vi "simple_loop.vi"() -> ()   [LabVIEW 2023]
panel:
  out "Numeric 3":i32
  in  "Numeric 2":i32
  out "Numeric":i32
  in  "max number of loop":i32
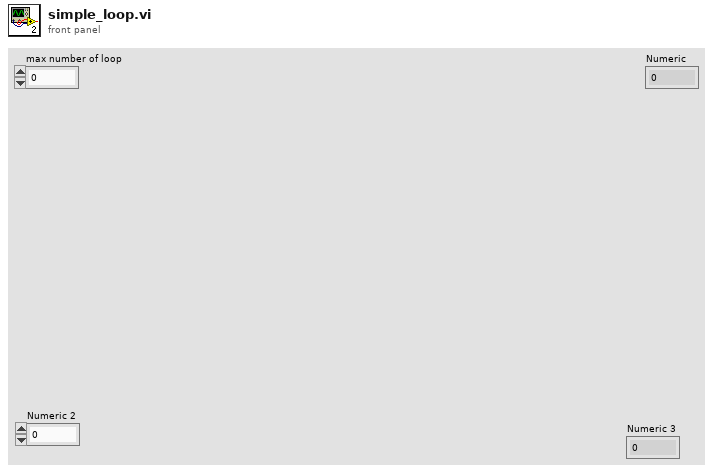
[diagram p1: front panel]
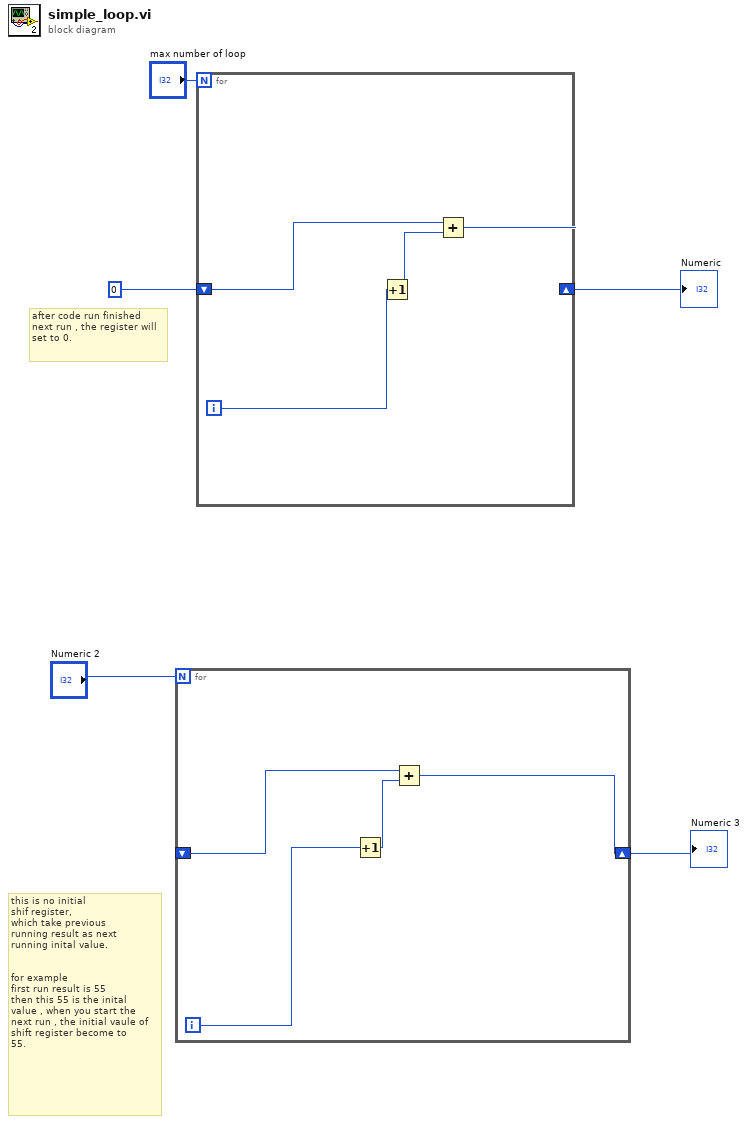
[diagram p0: block diagram]
diagram:
  # "after code run finished \nnext run , the register will\nset to 0."
  # "this is no initial\nshif register,\nwhich take previous\nrunning result as next \nrunning inital value.\n\n\nfor example \nfirst run result is 55 \nthen this 55 is the inital\nvalue , when you start the \nnext run , the initial vaule of \nshift register become to \n55."
  n1 = for {
    N: "Numeric 2" -> [_]
    shift-right: [w6] -> w1
    shift-left: _ -> [w7]
    i -> [w9]
    n2 = Increment(x=w9) -> (x+1=w8:i32)
    n3 = Add(x=w7, y=w8) -> (x+y=w6:i32)
  }
  "Numeric 3" <- w1
  n4 = for {
    N: "max number of loop" -> [_]
    shift-right: [w12] -> w4
    shift-left: 0 -> [w10]
    i -> [w13]
    n5 = Increment(x=w13) -> (x+1=w11:i32)
    n6 = Add(x=w10, y=w11) -> (x+y=w12:i32)
  }
  "Numeric" <- w4
